vi "ControlCenter.vi"() -> ()   [LabVIEW 2017]
uses:
  <vilib>/myRIO/Common/Instrument Driver Framework/myRIO v1.0/UART/vis/myRIO v1.0 Close UART.vi
  <vilib>/myRIO/Common/Instrument Driver Framework/Utilities/vis/FPGA Ref Manager.vi
  <vilib>/myRIO/Common/Instrument Driver Framework/myRIO v1.0/myRIO v1.0 Reset FPGA.vi
  <vilib>/myRIO/Common/Instrument Driver Framework/myRIO v1.0/IRQ/vis/myRIO v1.0 IRQ Info FGV.vi
  <vilib>/myRIO/Common/Instrument Driver Framework/myRIO v1.0/IRQ/vis/myRIO v1.0 Timer IRQ Info FGV.vi
  <vilib>/myRIO/Common/Instrument Driver Framework/myRIO v1.0/IRQ/vis/myRIO v1.0 ISR Agent.vi
  <vilib>/myRIO/Instrument Drivers/Utilities/Utilities.lvlib
panel:
  out "iterationaccel":i32
  out "y":dbl(graph)
  out "z":dbl(graph)
  out "x\nx":dbl(graph)
  out "Zaxis":dbl
  out "Yaxis":dbl
  out "Xaxis":dbl
  out "LonDeg":dbl format="%.6g"
  out "latDeg":dbl format="%.6g"
  out "Sat 2":i32
  out "Key Number":i16
  in  "MODE":bool
  out "Longitude":dbl(graph)
  out "Latitude":dbl(graph)
  out "Sat":i32(graph)
  out "ReadMe":string
  out "Battery Level":dbl(slide) scale=8.5..12.0 scale format="%#_4g"
  out "iteration":i32
  out "iteration":i32
  out "iteration":i32
  out "iteration":i32
  out "iteration":i32
  out "Right":dbl format="%#_4g"
  out "Right":dbl
  out "Left":dbl format="%#_4g"
  out "Left":dbl
  out "Speed-R":i8(slide) min=-100 max=100 step=1 scale=-100.0..100.0
  out "Speed-L":i8(slide) min=-100 max=100 step=1 scale=-100.0..100.0
  in  "stop":bool
  out "Particle (x,y,pixels)":dbl[][](array[numeric]) format="%_2f"
  out "Acquired\nFrames/s":dbl format="%.1g"
  in  "Decoration":bool
  in  "Decoration 2":bool
  in  "Decoration 3":bool
  in  "Decoration 4":bool
  in  "Decoration 5":bool
  in  "Decoration 6":bool
  # "ASEP Robot Control"
  # "Vision Control"
  # "Motor Driver Data"
  # "GPS Data"
  # "Motor Control"
  # "Keyboard and XYZ"
  # "Temp (C)"
  # "Voltage (v)"
  # "Battery Level (v)"
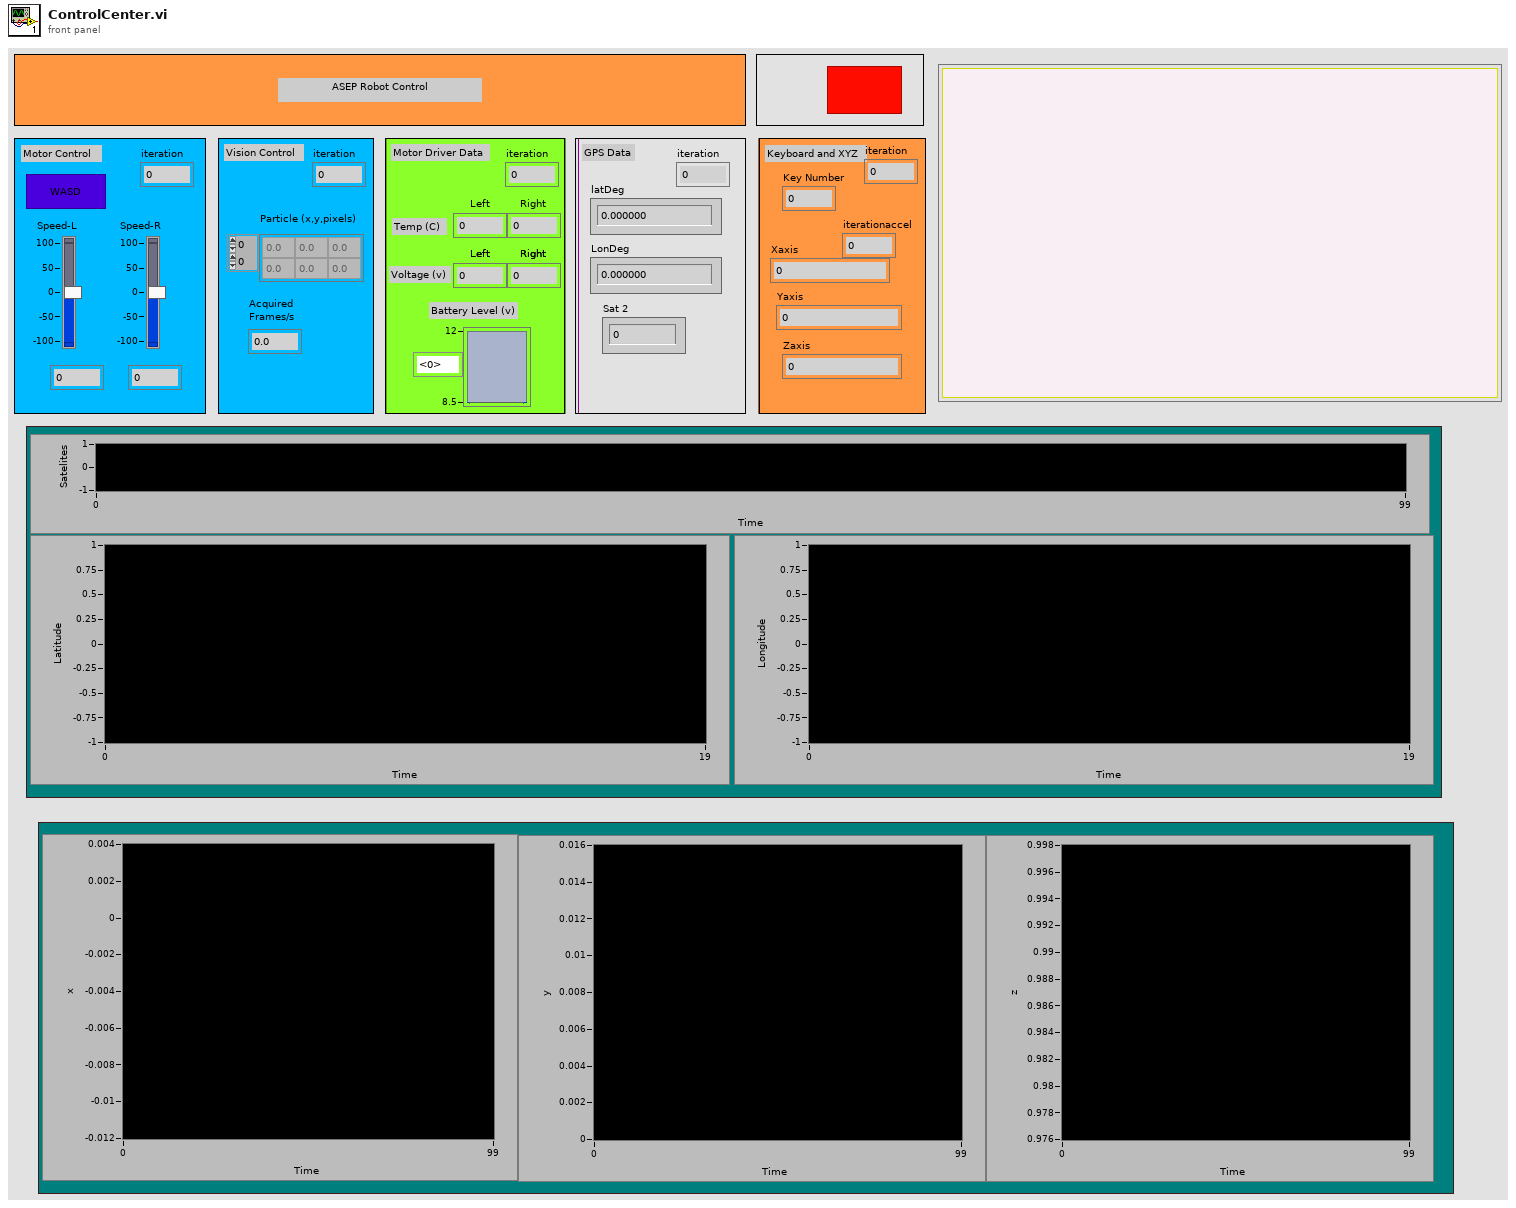
[diagram p1: front panel]
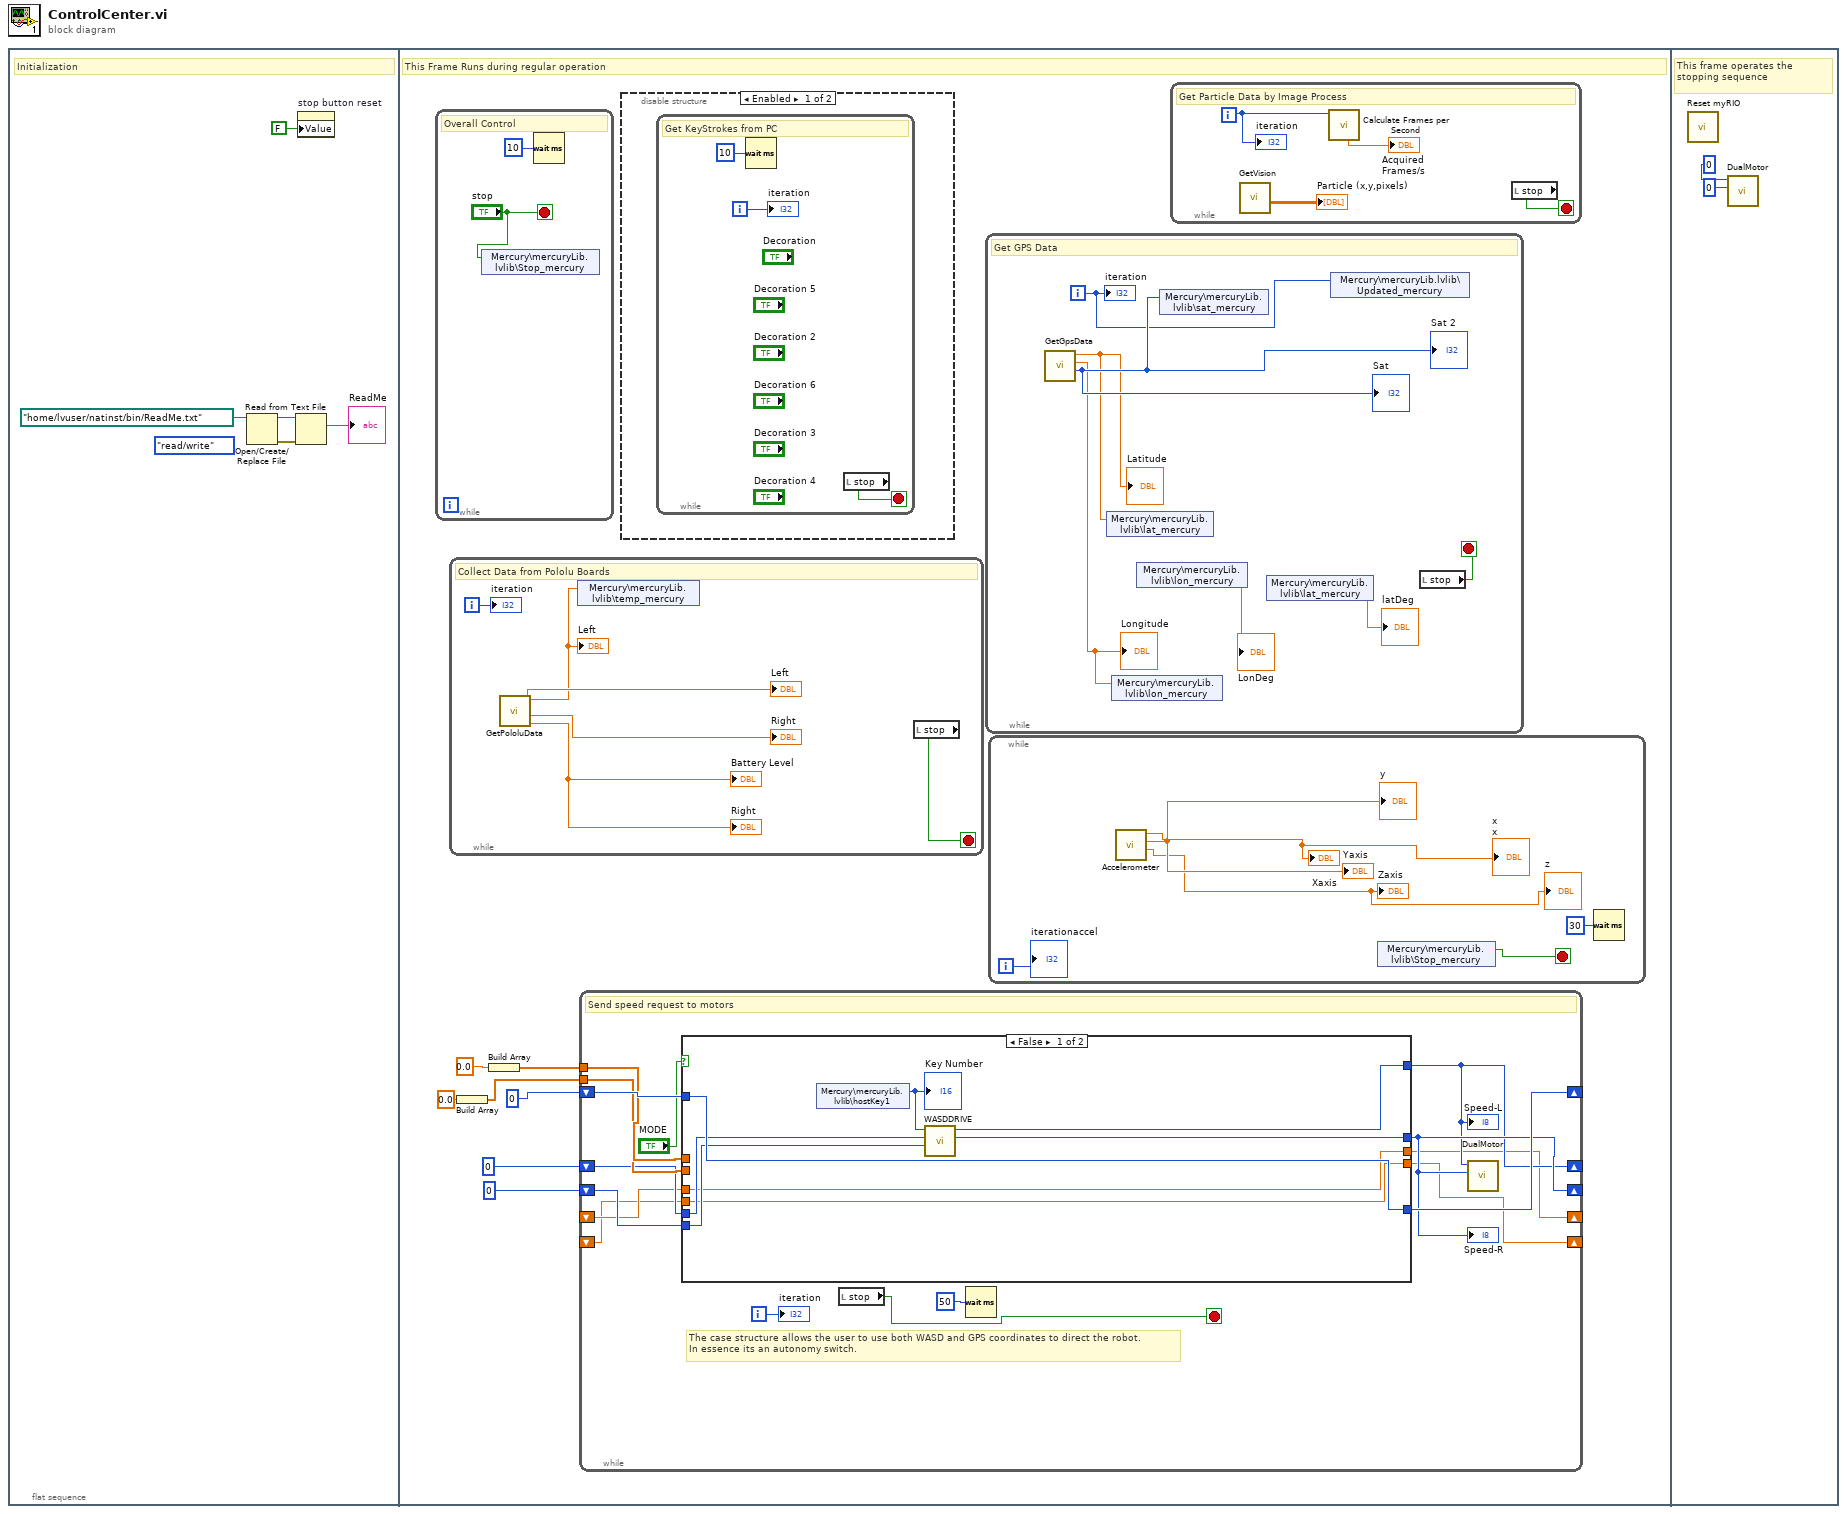
[diagram p0: block diagram]
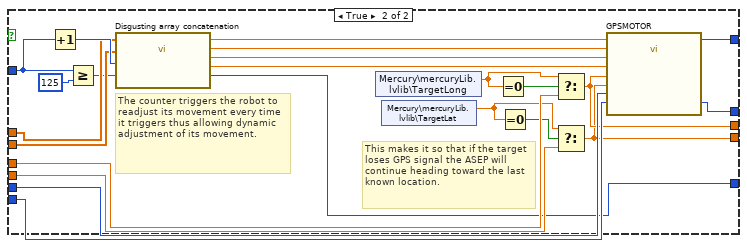
[diagram p3: hidden frame]
diagram:
  n1 = flat-sequence {
    frame #0 {
      (unwired) enum16{"read/write", "read-only", "write-only"}."read/write" ("access (0:read/write)")
      # "Initialization"
      n2 = Open/Create/Replace File(file path (use dialog)=path "/home/lvuser/natinst/bin/ReadMe.txt" ("file (use dialog)")) -> (refnum out=w3:refnum<file>, error out=w4:errorcluster)  [unwired: 5 in, 1 out]
      n3 = Read from Text File(file (use dialog)=w3, error in=w4) -> (text=→"ReadMe":string)  [unwired: 2 in, 3 out]
      n4 = property on="stop button reset" class="Bool (strict)"("Value"=FALSE ("stop")) -> ()  [unwired: 2 in, 2 out]
    }
    frame #1 {
      # "This Frame Runs during regular operation"
      n5 = while {
        stop <- "stop" stop-if-true
        # "Overall Control"
        n6 = shared-variable "Mercury\\mercuryLib.lvlib\\Stop_mercury"("stop") -> ()  [unwired: 1 in, 1 out]
        n7 = Wait (ms)(milliseconds to wait=u32 10) -> ()  [unwired: 1 out]
      }
      n8 = while {
        i -> [w36]
        stop <- w38 stop-if-true
        # "Collect Data from Pololu Boards"
        n9 = call "GetPololuData.vi"() -> ("Right Board Voltage"=→"Right" →"Battery Level":dbl, "Right Board Temp"=→"Right":dbl, "Left Board Voltage"=→"Left":dbl, "Left Board Temp"=w37:dbl)  [unwired: 8 in]
        "Left" <- w37
        n10 = shared-variable "Mercury\\mercuryLib.lvlib\\temp_mercury"(w37) -> ()  [unwired: 1 in, 1 out]
        n11 = local read "stop"() -> (w38:bool)
        "iteration" <- w36
      }
      n12 = Build Array(0.0 ("element")) -> (w8:dbl[])
      n13 = Build Array(0.0 ("element")) -> (w11:dbl[])
      n14 = while {
        shift-right: [w54] -> _
        shift-left: u32 0 ("milliseconds to wait") -> [w55]
        shift-right: [w47] -> _
        shift-left: i8 0 ("LeftOUT") -> [w51]
        shift-right: [w48] -> _
        shift-left: i8 0 ("RightOUT") -> [w50]
        tunnel: w11 -> [w53]
        tunnel: w8 -> [w52]
        shift-right: [w45] -> _
        shift-left: _ -> [w46]
        shift-right: [w43] -> _
        shift-left: _ -> [w44]
        i -> [w41]
        stop <- w42 stop-if-true
        # "The case structure allows the user to use both WASD and GPS coordinates to direct the robot.\nIn essence its an autonomy switch."
        # "Send speed request to motors"
        n15 = case shown="False" "MODE" {
          tunnel: w55 -> [w64 w86]
          tunnel: [w64 w65] -> w54
          tunnel: w53 -> [_ w84]
          tunnel: w52 -> [_ w83]
          tunnel: [w59 w78] -> w48
          tunnel: [w60 w79] -> w47
          tunnel: w51 -> [w62 w82]
          tunnel: w50 -> [w61 w81]
          tunnel: w46 -> [w58 w73]
          tunnel: [w58 w72] -> w45
          tunnel: w44 -> [w57 w67]
          tunnel: [w57 w66] -> w43
          frame False {
            n16 = shared-variable "Mercury\\mercuryLib.lvlib\\hostKey1"() -> (w63:i16)  [unwired: 1 in, 1 out]
            "Key Number" <- w63
            n17 = call "WASDDRIVE.vi"("RIGHTIN"=w61, "LEFTIN"=w62, "KEY"=w63) -> ("RIGHTOUT"=w59:i8, "LEFTOUT"=w60:i8)  [unwired: 7 in]
          }
          frame True {
            # "This makes it so that if the target loses GPS signal the ASEP will continue heading toward the last known location."
            # "The counter triggers the robot to readjust its movement every time it triggers thus allowing dynamic adjustment of its movement."
            n18 = Increment(x=w86) -> (x+1=w85:u32)
            n19 = Greater Or Equal?(x=w86, y=125) -> (x >= y?=w80:bool)
            n20 = call "Disgusting array concatenation.vi"("Trigger"=w80, "COUNTIN"=w85, "LongitudeArray"=w83, "LatitudeArray"=w84) -> ("CurrentLon"=w74:dbl, "CurrentLat"=w75:dbl, "PastLon"=w76:dbl, "PastLat"=w77:dbl, "COUNTOUT"=w65:u32)  [unwired: 3 in]
            n21 = shared-variable "Mercury\\mercuryLib.lvlib\\TargetLong"() -> (w70:dbl)  [unwired: 1 in, 1 out]
            n22 = shared-variable "Mercury\\mercuryLib.lvlib\\TargetLat"() -> (w69:dbl)  [unwired: 1 in, 1 out]
            n23 = Equal To 0?(x=w70) -> (x = 0?=w71:bool)
            n24 = Equal To 0?(x=w69) -> (x = 0?=w68:bool)
            n25 = Select(t=w70, s=w71, f=w73) -> (s? t:f=w72:dbl)
            n26 = Select(t=w69, s=w68, f=w67) -> (s? t:f=w66:dbl)
            n27 = call "GPSMOTOR.vi"("PastLat"=w77, "PastLon"=w76, "CurrentLat"=w75, "CurrentLon"=w74, "TargetLong"=w72, "TargetLat"=w66, "LeftIN"=w82, "RightIN"=w81) -> ("LeftOUT"=w79:i8, "RightOUT"=w78:i8)  [unwired: 18 in]
          }
        }
        "Speed-L" <- w47
        "Speed-R" <- w48
        n28 = local read "stop"() -> (w42:bool)
        n29 = Wait (ms)(milliseconds to wait=u32 50) -> ()  [unwired: 1 out]
        n30 = call "DualMotor.vi"("Speed-R"=w48, "Speed-L"=w47) -> ()  [unwired: 10 in]
        "iteration" <- w41
      }
      n31 = disable-structure shown="Enabled" {
        frame Enabled {
          n32 = while {
            i -> [w24]
            stop <- w25 stop-if-true
            # "Get KeyStrokes from PC"
            n33 = Wait (ms)(milliseconds to wait=u32 10) -> ()  [unwired: 1 out]
            n34 = local read "stop"() -> (w25:bool)
            "iteration" <- w24
          }
        }
        frame Disabled {
        }
      }
      n35 = while {
        i -> [w28]
        stop <- w29 stop-if-true
        # "Get GPS Data"
        n36 = call "GetGpsData.vi"() -> ("latDeg"=w31:dbl, "LonDeg"=w30:dbl, "Sat"=w32:i32)  [unwired: 7 in]
        "Sat" <- w32
        "Latitude" <- w31
        "Longitude" <- w30
        "Sat 2" <- w32
        n37 = shared-variable "Mercury\\mercuryLib.lvlib\\lat_mercury"(w31) -> ()  [unwired: 1 in, 1 out]
        n38 = shared-variable "Mercury\\mercuryLib.lvlib\\lon_mercury"(w30) -> ()  [unwired: 1 in, 1 out]
        n39 = shared-variable "Mercury\\mercuryLib.lvlib\\lon_mercury"() -> (→"LonDeg":dbl)  [unwired: 1 in, 1 out]
        n40 = shared-variable "Mercury\\mercuryLib.lvlib\\sat_mercury"(w32) -> ()  [unwired: 1 in, 1 out]
        n41 = shared-variable "Mercury\\mercuryLib.lvlib\\lat_mercury"() -> (→"latDeg":dbl)  [unwired: 1 in, 1 out]
        n42 = shared-variable "Mercury\\mercuryLib.lvlib\\Updated_mercury"(w28) -> ()  [unwired: 1 in, 1 out]
        n43 = local read "stop"() -> (w29:bool)
        "iteration" <- w28
      }
      n44 = while {
        i -> [w16]
        stop <- w18 stop-if-true
        n45 = call "Accelerometer.vi"() -> ("Z-Axis"=→"Zaxis" →"z":dbl, "Y-Axis"=→"Yaxis" →"y":dbl, "X-Axis"=→"Xaxis" →"x\nx":dbl)  [unwired: 9 in]
        n46 = shared-variable "Mercury\\mercuryLib.lvlib\\Stop_mercury"() -> (w18:bool)  [unwired: 1 in, 1 out]
        n47 = Wait (ms)(milliseconds to wait=u32 30) -> ()  [unwired: 1 out]
        "iterationaccel" <- w16
      }
      n48 = while {
        i -> [w21]
        stop <- w19 stop-if-true
        # "Get Particle Data by Image Process"
        n49 = call "GetVision.vi"() -> ("Particle Measurements\n         X             Y           area"=→"Particle (x,y,pixels)":dbl[][])  [unwired: 11 in]
        n50 = call <vilib>:"Calculate Frames per Second.vi"("Buffer Number"=w21) -> ("Acquired Frames/s"=→"Acquired\nFrames/s":dbl)  [unwired: 8 in, 2 out]
        n51 = local read "stop"() -> (w19:bool)
        "iteration" <- w21
      }
    }
    frame #2 {
      # "This frame operates the stopping sequence"
      n52 = call <vilib>:"Reset myRIO.vi"() -> ()  [unwired: 11 in, 1 out]
      n53 = call "DualMotor.vi"("Speed-R"=i8 0 ("Speed-R 2"), "Speed-L"=i8 0 ("Speed-L 2")) -> ()  [unwired: 10 in]
    }
  }
